vi "GDX_GetSensorInfo.vi"() -> (2 "battery level":u8)   [LabVIEW 2019]
uses:
  <vilib>/Vernier/GDX/GDX Controls/D2PIO_CHARGER_STATE.ctl
panel:
  out "Channel 15":i8
  out "Ch is Active 15":bool
  out "Channel Unit 15":string
  out "Channel Description 15":string
  out "Channel 14":i8
  out "Ch is Active 14":bool
  out "Channel Unit 14":string
  out "Channel Description 14":string
  out "Channel 13":i8
  out "Ch is Active 13":bool
  out "Channel Unit 13":string
  out "Channel Description 13":string
  out "Channel 12":i8
  out "Ch is Active 12":bool
  out "Channel Unit 12":string
  out "Channel Description 12":string
  out "Channel 11":i8
  out "Ch is Active 11":bool
  out "Channel Unit 11":string
  out "Channel Description 11":string
  out "Channel 10":i8
  out "Ch is Active 10":bool
  out "Channel Unit 10":string
  out "Channel Description 10":string
  out "Channel 9":i8
  out "Ch is Active 9":bool
  out "Channel Unit 9":string
  out "Channel Description 9":string
  out "Channel 8":i8
  out "Ch is Active 8":bool
  out "Channel Unit 8":string
  out "Channel Description 8":string
  out "Channel 7":i8
  out "Ch is Active 7":bool
  out "Channel Unit 7":string
  out "Channel Description 7":string
  out "Channel 6":i8
  out "Ch is Active 6":bool
  out "Channel Unit 6":string
  out "Channel Description 6":string
  out "Channel 5":i8
  out "Ch is Active 5":bool
  out "Channel Unit 5":string
  out "Channel Description 5":string
  out "Channel 4":i8
  out "Ch is Active 4":bool
  out "Channel Unit 4":string
  out "Channel Description 4":string
  out "Channel 3":i8
  out "Ch is Active 3":bool
  out "Channel Unit 3":string
  out "Channel Description 3":string
  out "Channel Unit 2":string
  out "Channel Description 2":string
  out "Ch is Active 2":bool
  out "Channel 2":i8
  out "Channel Unit":string
  out "Channel Description":string
  out "Ch is Active":bool
  out "Channel":i8
  out "BT Address (hex string)":string
  out "BLE Firmware (Numeric)":dbl
  out "DAQ Firmware (Numeric)":dbl
  out "Day":u8
  out "Month":u8
  out "Year":u16
  out "Device Name":string
  out "Device Friendly Name":string
  out "Serial Number":string
  out "Order Code":string
  out "CHARGER_STATE":T1 items=["IDLE", "CHARGING", "COMPLETE", "ERROR"]
  out "Available Channels":i8[](array[numeric])
  out "error out":errorcluster
  # "CHANNEL INFORMATION"
  # "DEVICE INFORMATION"
  # "Channel"
  # "Active?"
  # "Description"
  # "Unit"
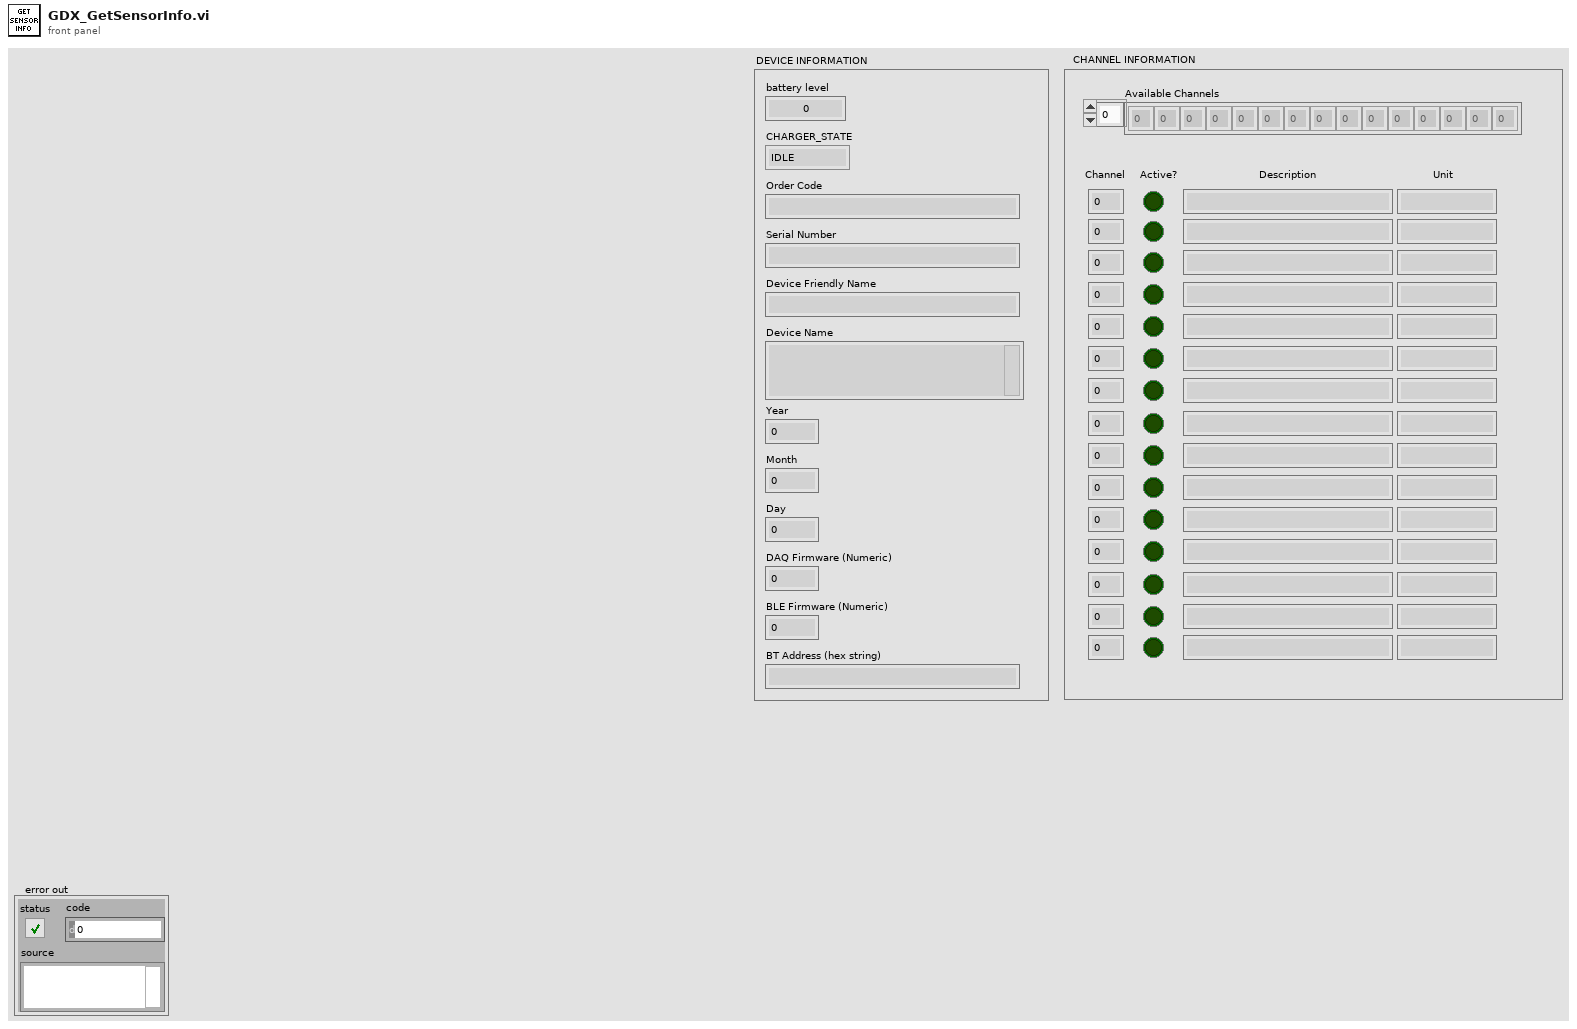
[diagram p1: front panel]
types:
  T1 = typedef "D2PIO_CHARGER_STATE.ctl" = u8
  T2 = typedef "D2PIO_D2PIOCluster.ctl" = cluster{"Library Handle":i64, "Device List Handle":i64, "BT Device Handles":i64[], "USB Device Handles":i64[], "BT+USB Device Handles":i64[], "Measurement Tick":dbl[], "Ch Availability Mask":u32[]}
  T3 = typedef "D2PIO_ChannelInfoCluster.ctl" = cluster{"Channel":i8, "Ch is Active":bool, "Channel ID":u32, "Channel Description":string, "Channel Unit":string}[]
  T4 = typedef "D2PIO_INFO_DeviceInfoCluster.ctl" = cluster{"battery level":u8, "CHARGER_STATE":T1, "Order Code":string, "Serial Number":string, "MFG ID":i16, "Device Friendly Name":string, "Device Name":string, "Year":u16, "Month":u8, "Day":u8, "DAQ Firmware (Numeric)":dbl, "DAQ Firmware (String)":string, "BLE Firmware (Numeric)":dbl, "BLE Firmware (String)":string, "BT Address (hex string)":string}
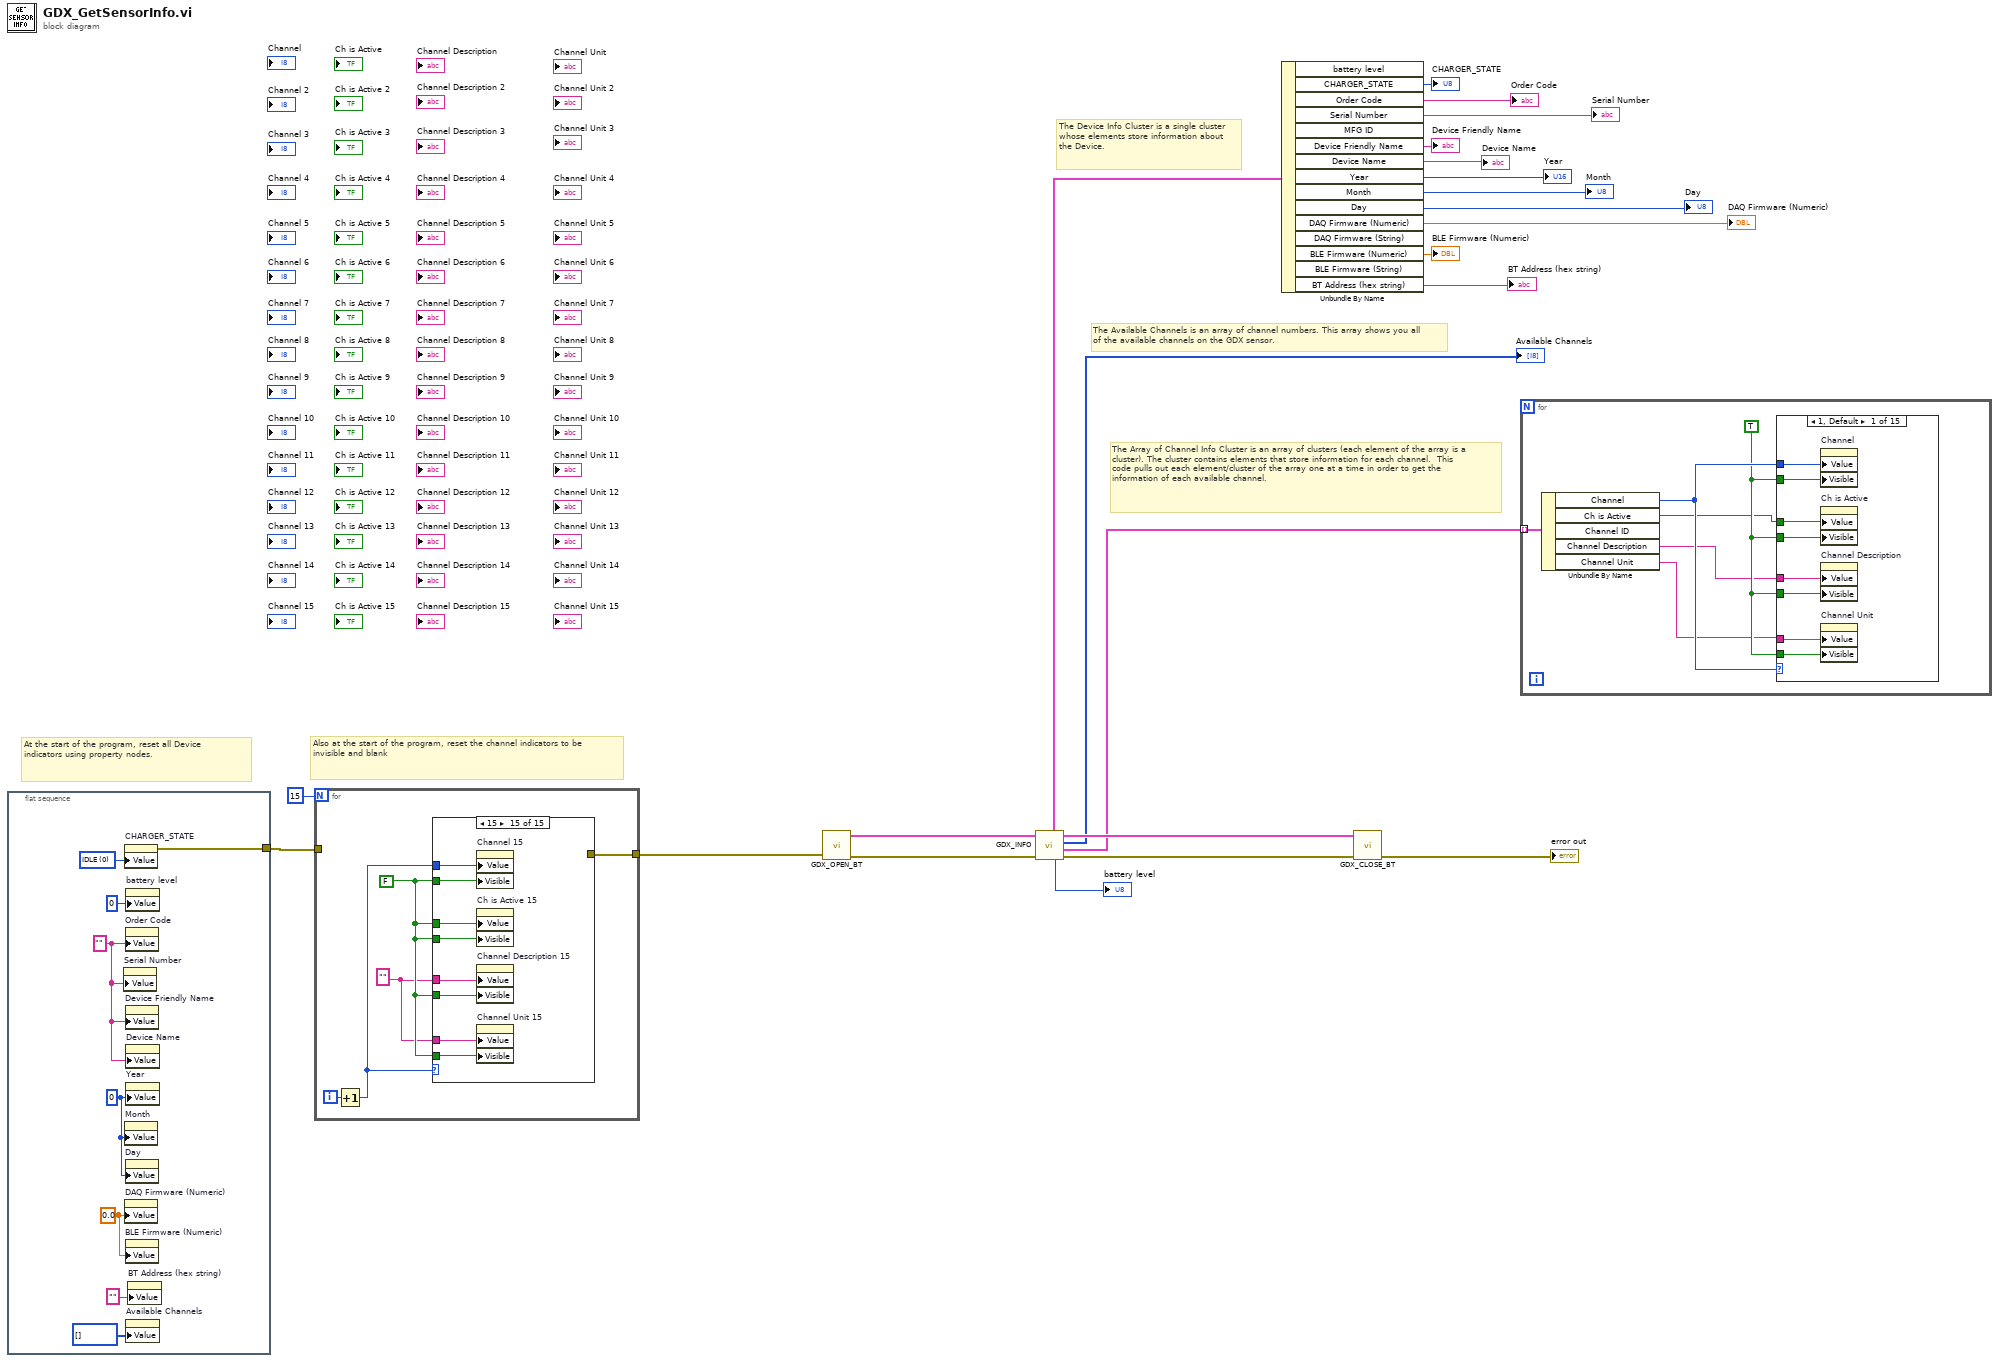
[diagram p0: block diagram]
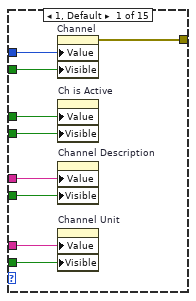
[diagram p2: hidden frame]
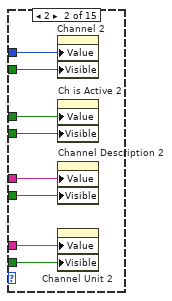
[diagram p3: hidden frame]
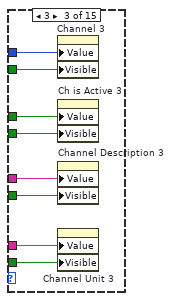
[diagram p4: hidden frame]
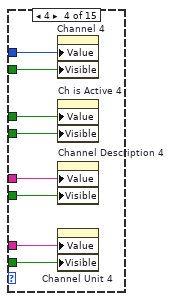
[diagram p5: hidden frame]
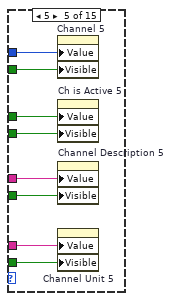
[diagram p6: hidden frame]
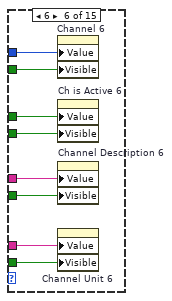
[diagram p7: hidden frame]
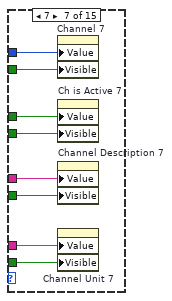
[diagram p8: hidden frame]
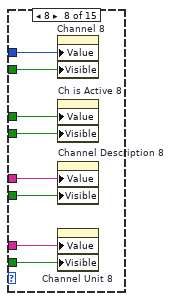
[diagram p9: hidden frame]
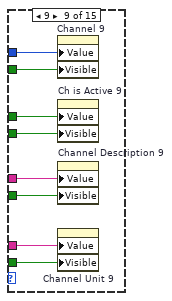
[diagram p10: hidden frame]
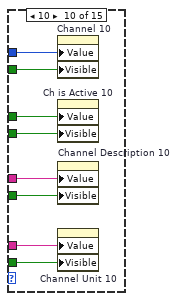
[diagram p11: hidden frame]
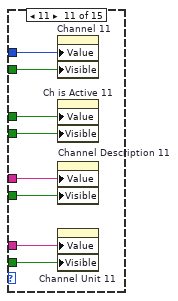
[diagram p12: hidden frame]
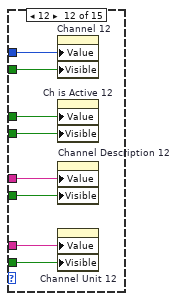
[diagram p13: hidden frame]
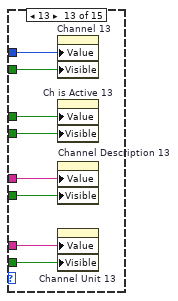
[diagram p14: hidden frame]
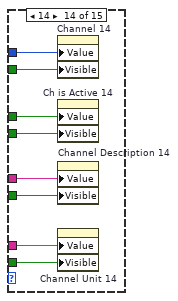
[diagram p15: hidden frame]
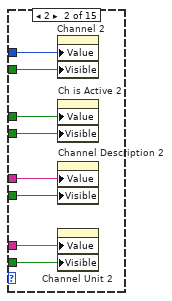
[diagram p16: hidden frame]
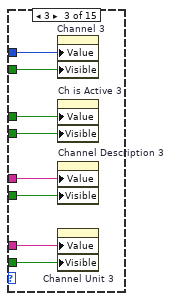
[diagram p17: hidden frame]
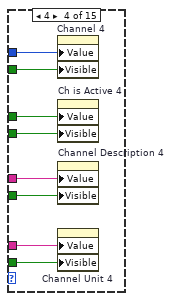
[diagram p18: hidden frame]
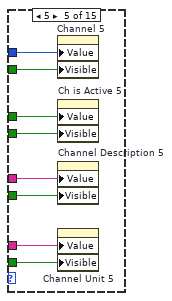
[diagram p19: hidden frame]
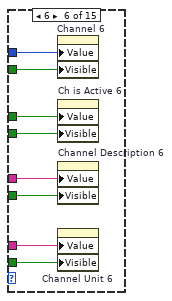
[diagram p20: hidden frame]
diagram:
  # "The Available Channels is an array of channel numbers. This array shows you all of the available channels on the GDX sensor."
  # "The Device Info Cluster is a single cluster whose elements store information about the Device."
  # "At the start of the program, reset all Device indicators using property nodes."
  # "The Array of Channel Info Cluster is an array of clusters (each element of the array is a cluster). The cluster contains elements that store information for each channel.  This code pulls out each element/cluster of the array one at a time in order to get the information of each available channel."
  # "Also at the start of the program, reset the channel indicators to be invisible and blank"
  n1 = flat-sequence {
    tunnel: [w25] -> w1
    frame #0 {
      w28 = 0.0 ("DAQ Firmware (Numeric)")
      w29 = u16 0 ("Year")
      w30 = "" ("Order Code")
      w31 = T1 0 items=["IDLE", "CHARGING", "COMPLETE", "ERROR"] ("CHARGER_STATE")
      n2 = property on="Serial Number" class="Str"("Value"=w30) -> ()  [unwired: 2 in, 2 out]
      n3 = property on="CHARGER_STATE" class="Ring (strict)"("Value"=w31) -> (error out=w25:errorcluster)  [unwired: 2 in, 1 out]
      n4 = property on="Month" class="DigNum (strict)"("Value"=w29) -> ()  [unwired: 2 in, 2 out]
      n5 = property on="DAQ Firmware (Numeric)" class="DigNum (strict)"("Value"=w28) -> ()  [unwired: 2 in, 2 out]
      n6 = property on="Order Code" class="Str"("Value"=w30) -> ()  [unwired: 2 in, 2 out]
      n7 = property on="Device Friendly Name" class="Str"("Value"=w30) -> ()  [unwired: 2 in, 2 out]
      n8 = property on="Day" class="DigNum (strict)"("Value"=w29) -> ()  [unwired: 2 in, 2 out]
      n9 = property on="BLE Firmware (Numeric)" class="DigNum (strict)"("Value"=w28) -> ()  [unwired: 2 in, 2 out]
      n10 = property on="battery level" class="DigNum (strict)"("Value"=u8 0 ("battery level")) -> ()  [unwired: 2 in, 2 out]
      n11 = property on="Device Name" class="Str"("Value"=w30) -> ()  [unwired: 2 in, 2 out]
      n12 = property on="Year" class="DigNum (strict)"("Value"=w29) -> ()  [unwired: 2 in, 2 out]
      n13 = property on="Available Channels" class="Arr (strict)"("Value"=i8[] [] ("Available Channels")) -> ()  [unwired: 2 in, 2 out]
      n14 = property on="BT Address (hex string)" class="Str"("Value"="" ("BT Address (hex string)")) -> ()  [unwired: 2 in, 2 out]
    }
  }
  n15 = for {
    N: 15 -> [_]
    tunnel: [w33] -> w2
    tunnel: w1 -> [_]
    i -> [w36]
    w34 = "" ("Channel Description")
    w35 = FALSE ("Visible")
    n16 = Increment(x=w36) -> (x+1=w32:i32)
    n17 = case shown="15" w32 {
      tunnel: w32 -> [w45 w53 w61 w69 w77 w85 w93 w101 w109 w117 w125 w133 w141 w149 w157]
      tunnel: w35 -> [w44 w52 w60 w68 w76 w84 w92 w100 w108 w116 w124 w132 w140 w148 w156]
      tunnel: w35 -> [w43 w51 w59 w67 w75 w83 w91 w99 w107 w115 w123 w131 w139 w147 w155]
      tunnel: w35 -> [w42 w50 w58 w66 w74 w82 w90 w98 w106 w114 w122 w130 w138 w146 w154]
      tunnel: w35 -> [w41 w49 w57 w65 w73 w81 w89 w97 w105 w113 w121 w129 w137 w145 w153]
      tunnel: w35 -> [w40 w48 w56 w64 w72 w80 w88 w96 w104 w112 w120 w128 w136 w144 w152]
      tunnel: w34 -> [w39 w47 w55 w63 w71 w79 w87 w95 w103 w111 w119 w127 w135 w143 w151]
      tunnel: w34 -> [w38 w46 w54 w62 w70 w78 w86 w94 w102 w110 w118 w126 w134 w142 w150]
      tunnel: [w37 _ _ _ _ _ _ _ _ _ _ _ _ _ _] -> w33
      frame 1, Default {
        n18 = property on="Channel" class="DigNum (strict)"("Value"=w45, "Visible"=w44) -> (error out=w37:errorcluster)  [unwired: 2 in, 1 out]
        n19 = property on="Ch is Active" class="Bool (strict)"("Value"=w40, "Visible"=w43) -> ()  [unwired: 2 in, 2 out]
        n20 = property on="Channel Description" class="Str"("Value"=w39, "Visible"=w42) -> ()  [unwired: 2 in, 2 out]
        n21 = property on="Channel Unit" class="Str"("Value"=w38, "Visible"=w41) -> ()  [unwired: 2 in, 2 out]
      }
      frame 2 {
        n22 = property on="Channel 2" class="DigNum (strict)"("Value"=w53, "Visible"=w52) -> ()  [unwired: 2 in, 2 out]
        n23 = property on="Ch is Active 2" class="Bool (strict)"("Value"=w48, "Visible"=w51) -> ()  [unwired: 2 in, 2 out]
        n24 = property on="Channel Description 2" class="Str"("Value"=w47, "Visible"=w50) -> ()  [unwired: 2 in, 2 out]
        n25 = property on="Channel Unit 2" class="Str"("Value"=w46, "Visible"=w49) -> ()  [unwired: 2 in, 2 out]
      }
      frame 3 {
        n26 = property on="Channel 3" class="DigNum (strict)"("Value"=w61, "Visible"=w60) -> ()  [unwired: 2 in, 2 out]
        n27 = property on="Ch is Active 3" class="Bool (strict)"("Value"=w56, "Visible"=w59) -> ()  [unwired: 2 in, 2 out]
        n28 = property on="Channel Description 3" class="Str"("Value"=w55, "Visible"=w58) -> ()  [unwired: 2 in, 2 out]
        n29 = property on="Channel Unit 3" class="Str"("Value"=w54, "Visible"=w57) -> ()  [unwired: 2 in, 2 out]
      }
      frame 4 {
        n30 = property on="Channel 4" class="DigNum (strict)"("Value"=w69, "Visible"=w68) -> ()  [unwired: 2 in, 2 out]
        n31 = property on="Ch is Active 4" class="Bool (strict)"("Value"=w64, "Visible"=w67) -> ()  [unwired: 2 in, 2 out]
        n32 = property on="Channel Description 4" class="Str"("Value"=w63, "Visible"=w66) -> ()  [unwired: 2 in, 2 out]
        n33 = property on="Channel Unit 4" class="Str"("Value"=w62, "Visible"=w65) -> ()  [unwired: 2 in, 2 out]
      }
      frame 5 {
        n34 = property on="Channel 5" class="DigNum (strict)"("Value"=w77, "Visible"=w76) -> ()  [unwired: 2 in, 2 out]
        n35 = property on="Ch is Active 5" class="Bool (strict)"("Value"=w72, "Visible"=w75) -> ()  [unwired: 2 in, 2 out]
        n36 = property on="Channel Description 5" class="Str"("Value"=w71, "Visible"=w74) -> ()  [unwired: 2 in, 2 out]
        n37 = property on="Channel Unit 5" class="Str"("Value"=w70, "Visible"=w73) -> ()  [unwired: 2 in, 2 out]
      }
      frame 6 {
        n38 = property on="Channel 6" class="DigNum (strict)"("Value"=w85, "Visible"=w84) -> ()  [unwired: 2 in, 2 out]
        n39 = property on="Ch is Active 6" class="Bool (strict)"("Value"=w80, "Visible"=w83) -> ()  [unwired: 2 in, 2 out]
        n40 = property on="Channel Description 6" class="Str"("Value"=w79, "Visible"=w82) -> ()  [unwired: 2 in, 2 out]
        n41 = property on="Channel Unit 6" class="Str"("Value"=w78, "Visible"=w81) -> ()  [unwired: 2 in, 2 out]
      }
      frame 7 {
        n42 = property on="Channel 7" class="DigNum (strict)"("Value"=w93, "Visible"=w92) -> ()  [unwired: 2 in, 2 out]
        n43 = property on="Ch is Active 7" class="Bool (strict)"("Value"=w88, "Visible"=w91) -> ()  [unwired: 2 in, 2 out]
        n44 = property on="Channel Description 7" class="Str"("Value"=w87, "Visible"=w90) -> ()  [unwired: 2 in, 2 out]
        n45 = property on="Channel Unit 7" class="Str"("Value"=w86, "Visible"=w89) -> ()  [unwired: 2 in, 2 out]
      }
      frame 8 {
        n46 = property on="Channel 8" class="DigNum (strict)"("Value"=w101, "Visible"=w100) -> ()  [unwired: 2 in, 2 out]
        n47 = property on="Ch is Active 8" class="Bool (strict)"("Value"=w96, "Visible"=w99) -> ()  [unwired: 2 in, 2 out]
        n48 = property on="Channel Description 8" class="Str"("Value"=w95, "Visible"=w98) -> ()  [unwired: 2 in, 2 out]
        n49 = property on="Channel Unit 8" class="Str"("Value"=w94, "Visible"=w97) -> ()  [unwired: 2 in, 2 out]
      }
      frame 9 {
        n50 = property on="Channel 9" class="DigNum (strict)"("Value"=w109, "Visible"=w108) -> ()  [unwired: 2 in, 2 out]
        n51 = property on="Ch is Active 9" class="Bool (strict)"("Value"=w104, "Visible"=w107) -> ()  [unwired: 2 in, 2 out]
        n52 = property on="Channel Description 9" class="Str"("Value"=w103, "Visible"=w106) -> ()  [unwired: 2 in, 2 out]
        n53 = property on="Channel Unit 9" class="Str"("Value"=w102, "Visible"=w105) -> ()  [unwired: 2 in, 2 out]
      }
      frame 10 {
        n54 = property on="Channel 10" class="DigNum (strict)"("Value"=w117, "Visible"=w116) -> ()  [unwired: 2 in, 2 out]
        n55 = property on="Ch is Active 10" class="Bool (strict)"("Value"=w112, "Visible"=w115) -> ()  [unwired: 2 in, 2 out]
        n56 = property on="Channel Description 10" class="Str"("Value"=w111, "Visible"=w114) -> ()  [unwired: 2 in, 2 out]
        n57 = property on="Channel Unit 10" class="Str"("Value"=w110, "Visible"=w113) -> ()  [unwired: 2 in, 2 out]
      }
      frame 11 {
        n58 = property on="Channel 11" class="DigNum (strict)"("Value"=w125, "Visible"=w124) -> ()  [unwired: 2 in, 2 out]
        n59 = property on="Ch is Active 11" class="Bool (strict)"("Value"=w120, "Visible"=w123) -> ()  [unwired: 2 in, 2 out]
        n60 = property on="Channel Description 11" class="Str"("Value"=w119, "Visible"=w122) -> ()  [unwired: 2 in, 2 out]
        n61 = property on="Channel Unit 11" class="Str"("Value"=w118, "Visible"=w121) -> ()  [unwired: 2 in, 2 out]
      }
      frame 12 {
        n62 = property on="Channel 12" class="DigNum (strict)"("Value"=w133, "Visible"=w132) -> ()  [unwired: 2 in, 2 out]
        n63 = property on="Ch is Active 12" class="Bool (strict)"("Value"=w128, "Visible"=w131) -> ()  [unwired: 2 in, 2 out]
        n64 = property on="Channel Description 12" class="Str"("Value"=w127, "Visible"=w130) -> ()  [unwired: 2 in, 2 out]
        n65 = property on="Channel Unit 12" class="Str"("Value"=w126, "Visible"=w129) -> ()  [unwired: 2 in, 2 out]
      }
      frame 13 {
        n66 = property on="Channel 13" class="DigNum (strict)"("Value"=w141, "Visible"=w140) -> ()  [unwired: 2 in, 2 out]
        n67 = property on="Ch is Active 13" class="Bool (strict)"("Value"=w136, "Visible"=w139) -> ()  [unwired: 2 in, 2 out]
        n68 = property on="Channel Description 13" class="Str"("Value"=w135, "Visible"=w138) -> ()  [unwired: 2 in, 2 out]
        n69 = property on="Channel Unit 13" class="Str"("Value"=w134, "Visible"=w137) -> ()  [unwired: 2 in, 2 out]
      }
      frame 14 {
        n70 = property on="Channel 14" class="DigNum (strict)"("Value"=w149, "Visible"=w148) -> ()  [unwired: 2 in, 2 out]
        n71 = property on="Ch is Active 14" class="Bool (strict)"("Value"=w144, "Visible"=w147) -> ()  [unwired: 2 in, 2 out]
        n72 = property on="Channel Description 14" class="Str"("Value"=w143, "Visible"=w146) -> ()  [unwired: 2 in, 2 out]
        n73 = property on="Channel Unit 14" class="Str"("Value"=w142, "Visible"=w145) -> ()  [unwired: 2 in, 2 out]
      }
      frame 15 {
        n74 = property on="Channel 15" class="DigNum (strict)"("Value"=w157, "Visible"=w156) -> ()  [unwired: 2 in, 2 out]
        n75 = property on="Ch is Active 15" class="Bool (strict)"("Value"=w152, "Visible"=w155) -> ()  [unwired: 2 in, 2 out]
        n76 = property on="Channel Description 15" class="Str"("Value"=w151, "Visible"=w154) -> ()  [unwired: 2 in, 2 out]
        n77 = property on="Channel Unit 15" class="Str"("Value"=w150, "Visible"=w153) -> ()  [unwired: 2 in, 2 out]
      }
    }
  }
  n78 = call <vilib>:"GDX_OPEN_BT.vi"("error in (no error)"=w2) -> ("error out"=w21:errorcluster, "D2PIO Cluster Out"=w22:T2)  [unwired: 9 in]
  n79 = call <vilib>:"GDX_INFO.vi"("error in (no error)"=w21, "D2PIO Cluster In"=w22) -> ("error out"=w19:errorcluster, "Array of Channel Info Cluster"=w4:T3, "Available Channels"=→"Available Channels":i8[], "D2PIO Cluster Out"=w20:T2, "battery level"=→"battery level":u8, "Device Info Cluster"=w16:T4)  [unwired: 4 in]
  n80 = Unbundle By Name(w16) -> ("CHARGER_STATE"=→"CHARGER_STATE":T1, "Order Code"=→"Order Code":string, "Serial Number"=→"Serial Number":string, "Device Friendly Name"=→"Device Friendly Name":string, "Device Name"=→"Device Name":string, "Year"=→"Year":u16, "Month"=→"Month":u8, "Day"=→"Day":u8, "DAQ Firmware (Numeric)"=→"DAQ Firmware (Numeric)":dbl, "BLE Firmware (Numeric)"=→"BLE Firmware (Numeric)":dbl, "BT Address (hex string)"=→"BT Address (hex string)":string)  [unwired: 4 out]
  n81 = call <vilib>:"GDX_CLOSE_BT.vi"("error in (no error)"=w19, "D2PIO Cluster In"=w20) -> ("error out"=→"error out":errorcluster)  [unwired: 8 in, 1 out]
  n82 = for {
    tunnel: w4 -> [w163] mode=indexing
    w161 = TRUE ("Visible")
    n83 = Unbundle By Name(w163) -> ("Channel"=w162:i8, "Ch is Active"=w160:bool, "Channel Description"=w159:string, "Channel Unit"=w158:string)  [unwired: 1 out]
    n84 = case shown="1, Default" w162 {
      tunnel: w162 -> [w171 w179 w187 w195 w203 w211 w219 w227 w235 w243 w251 w259 w267 w275 w283]
      tunnel: w161 -> [w170 w178 w186 w194 w202 w210 w218 w226 w234 w242 w250 w258 w266 w274 w282]
      tunnel: w161 -> [w169 w177 w185 w193 w201 w209 w217 w225 w233 w241 w249 w257 w265 w273 w281]
      tunnel: w161 -> [w168 w176 w184 w192 w200 w208 w216 w224 w232 w240 w248 w256 w264 w272 w280]
      tunnel: w161 -> [w167 w175 w183 w191 w199 w207 w215 w223 w231 w239 w247 w255 w263 w271 w279]
      tunnel: w160 -> [w166 w174 w182 w190 w198 w206 w214 w222 w230 w238 w246 w254 w262 w270 w278]
      tunnel: w159 -> [w165 w173 w181 w189 w197 w205 w213 w221 w229 w237 w245 w253 w261 w269 w277]
      tunnel: w158 -> [w164 w172 w180 w188 w196 w204 w212 w220 w228 w236 w244 w252 w260 w268 w276]
      frame 1, Default {
        n85 = property on="Channel" class="DigNum (strict)"("Value"=w171, "Visible"=w170) -> ()  [unwired: 2 in, 2 out]
        n86 = property on="Ch is Active" class="Bool (strict)"("Value"=w166, "Visible"=w169) -> ()  [unwired: 2 in, 2 out]
        n87 = property on="Channel Description" class="Str"("Value"=w165, "Visible"=w168) -> ()  [unwired: 2 in, 2 out]
        n88 = property on="Channel Unit" class="Str"("Value"=w164, "Visible"=w167) -> ()  [unwired: 2 in, 2 out]
      }
      frame 2 {
        n89 = property on="Channel 2" class="DigNum (strict)"("Value"=w179, "Visible"=w178) -> ()  [unwired: 2 in, 2 out]
        n90 = property on="Ch is Active 2" class="Bool (strict)"("Value"=w174, "Visible"=w177) -> ()  [unwired: 2 in, 2 out]
        n91 = property on="Channel Description 2" class="Str"("Value"=w173, "Visible"=w176) -> ()  [unwired: 2 in, 2 out]
        n92 = property on="Channel Unit 2" class="Str"("Value"=w172, "Visible"=w175) -> ()  [unwired: 2 in, 2 out]
      }
      frame 3 {
        n93 = property on="Channel 3" class="DigNum (strict)"("Value"=w187, "Visible"=w186) -> ()  [unwired: 2 in, 2 out]
        n94 = property on="Ch is Active 3" class="Bool (strict)"("Value"=w182, "Visible"=w185) -> ()  [unwired: 2 in, 2 out]
        n95 = property on="Channel Description 3" class="Str"("Value"=w181, "Visible"=w184) -> ()  [unwired: 2 in, 2 out]
        n96 = property on="Channel Unit 3" class="Str"("Value"=w180, "Visible"=w183) -> ()  [unwired: 2 in, 2 out]
      }
      frame 4 {
        n97 = property on="Channel 4" class="DigNum (strict)"("Value"=w195, "Visible"=w194) -> ()  [unwired: 2 in, 2 out]
        n98 = property on="Ch is Active 4" class="Bool (strict)"("Value"=w190, "Visible"=w193) -> ()  [unwired: 2 in, 2 out]
        n99 = property on="Channel Description 4" class="Str"("Value"=w189, "Visible"=w192) -> ()  [unwired: 2 in, 2 out]
        n100 = property on="Channel Unit 4" class="Str"("Value"=w188, "Visible"=w191) -> ()  [unwired: 2 in, 2 out]
      }
      frame 5 {
        n101 = property on="Channel 5" class="DigNum (strict)"("Value"=w203, "Visible"=w202) -> ()  [unwired: 2 in, 2 out]
        n102 = property on="Ch is Active 5" class="Bool (strict)"("Value"=w198, "Visible"=w201) -> ()  [unwired: 2 in, 2 out]
        n103 = property on="Channel Description 5" class="Str"("Value"=w197, "Visible"=w200) -> ()  [unwired: 2 in, 2 out]
        n104 = property on="Channel Unit 5" class="Str"("Value"=w196, "Visible"=w199) -> ()  [unwired: 2 in, 2 out]
      }
      frame 6 {
        n105 = property on="Channel 6" class="DigNum (strict)"("Value"=w211, "Visible"=w210) -> ()  [unwired: 2 in, 2 out]
        n106 = property on="Ch is Active 6" class="Bool (strict)"("Value"=w206, "Visible"=w209) -> ()  [unwired: 2 in, 2 out]
        n107 = property on="Channel Description 6" class="Str"("Value"=w205, "Visible"=w208) -> ()  [unwired: 2 in, 2 out]
        n108 = property on="Channel Unit 6" class="Str"("Value"=w204, "Visible"=w207) -> ()  [unwired: 2 in, 2 out]
      }
      frame 7 {
        n109 = property on="Channel 7" class="DigNum (strict)"("Value"=w219, "Visible"=w218) -> ()  [unwired: 2 in, 2 out]
        n110 = property on="Ch is Active 7" class="Bool (strict)"("Value"=w214, "Visible"=w217) -> ()  [unwired: 2 in, 2 out]
        n111 = property on="Channel Description 7" class="Str"("Value"=w213, "Visible"=w216) -> ()  [unwired: 2 in, 2 out]
        n112 = property on="Channel Unit 7" class="Str"("Value"=w212, "Visible"=w215) -> ()  [unwired: 2 in, 2 out]
      }
      frame 8 {
        n113 = property on="Channel 8" class="DigNum (strict)"("Value"=w227, "Visible"=w226) -> ()  [unwired: 2 in, 2 out]
        n114 = property on="Ch is Active 8" class="Bool (strict)"("Value"=w222, "Visible"=w225) -> ()  [unwired: 2 in, 2 out]
        n115 = property on="Channel Description 8" class="Str"("Value"=w221, "Visible"=w224) -> ()  [unwired: 2 in, 2 out]
        n116 = property on="Channel Unit 8" class="Str"("Value"=w220, "Visible"=w223) -> ()  [unwired: 2 in, 2 out]
      }
      frame 9 {
        n117 = property on="Channel 9" class="DigNum (strict)"("Value"=w235, "Visible"=w234) -> ()  [unwired: 2 in, 2 out]
        n118 = property on="Ch is Active 9" class="Bool (strict)"("Value"=w230, "Visible"=w233) -> ()  [unwired: 2 in, 2 out]
        n119 = property on="Channel Description 9" class="Str"("Value"=w229, "Visible"=w232) -> ()  [unwired: 2 in, 2 out]
        n120 = property on="Channel Unit 9" class="Str"("Value"=w228, "Visible"=w231) -> ()  [unwired: 2 in, 2 out]
      }
      frame 10 {
        n121 = property on="Channel 10" class="DigNum (strict)"("Value"=w243, "Visible"=w242) -> ()  [unwired: 2 in, 2 out]
        n122 = property on="Ch is Active 10" class="Bool (strict)"("Value"=w238, "Visible"=w241) -> ()  [unwired: 2 in, 2 out]
        n123 = property on="Channel Description 10" class="Str"("Value"=w237, "Visible"=w240) -> ()  [unwired: 2 in, 2 out]
        n124 = property on="Channel Unit 10" class="Str"("Value"=w236, "Visible"=w239) -> ()  [unwired: 2 in, 2 out]
      }
      frame 11 {
        n125 = property on="Channel 11" class="DigNum (strict)"("Value"=w251, "Visible"=w250) -> ()  [unwired: 2 in, 2 out]
        n126 = property on="Ch is Active 11" class="Bool (strict)"("Value"=w246, "Visible"=w249) -> ()  [unwired: 2 in, 2 out]
        n127 = property on="Channel Description 11" class="Str"("Value"=w245, "Visible"=w248) -> ()  [unwired: 2 in, 2 out]
        n128 = property on="Channel Unit 11" class="Str"("Value"=w244, "Visible"=w247) -> ()  [unwired: 2 in, 2 out]
      }
      frame 12 {
        n129 = property on="Channel 12" class="DigNum (strict)"("Value"=w259, "Visible"=w258) -> ()  [unwired: 2 in, 2 out]
        n130 = property on="Ch is Active 12" class="Bool (strict)"("Value"=w254, "Visible"=w257) -> ()  [unwired: 2 in, 2 out]
        n131 = property on="Channel Description 12" class="Str"("Value"=w253, "Visible"=w256) -> ()  [unwired: 2 in, 2 out]
        n132 = property on="Channel Unit 12" class="Str"("Value"=w252, "Visible"=w255) -> ()  [unwired: 2 in, 2 out]
      }
      frame 13 {
        n133 = property on="Channel 13" class="DigNum (strict)"("Value"=w267, "Visible"=w266) -> ()  [unwired: 2 in, 2 out]
        n134 = property on="Ch is Active 13" class="Bool (strict)"("Value"=w262, "Visible"=w265) -> ()  [unwired: 2 in, 2 out]
        n135 = property on="Channel Description 13" class="Str"("Value"=w261, "Visible"=w264) -> ()  [unwired: 2 in, 2 out]
        n136 = property on="Channel Unit 13" class="Str"("Value"=w260, "Visible"=w263) -> ()  [unwired: 2 in, 2 out]
      }
      frame 14 {
        n137 = property on="Channel 14" class="DigNum (strict)"("Value"=w275, "Visible"=w274) -> ()  [unwired: 2 in, 2 out]
        n138 = property on="Ch is Active 14" class="Bool (strict)"("Value"=w270, "Visible"=w273) -> ()  [unwired: 2 in, 2 out]
        n139 = property on="Channel Description 14" class="Str"("Value"=w269, "Visible"=w272) -> ()  [unwired: 2 in, 2 out]
        n140 = property on="Channel Unit 14" class="Str"("Value"=w268, "Visible"=w271) -> ()  [unwired: 2 in, 2 out]
      }
      frame 15 {
        n141 = property on="Channel 15" class="DigNum (strict)"("Value"=w283, "Visible"=w282) -> ()  [unwired: 2 in, 2 out]
        n142 = property on="Ch is Active 15" class="Bool (strict)"("Value"=w278, "Visible"=w281) -> ()  [unwired: 2 in, 2 out]
        n143 = property on="Channel Description 15" class="Str"("Value"=w277, "Visible"=w280) -> ()  [unwired: 2 in, 2 out]
        n144 = property on="Channel Unit 15" class="Str"("Value"=w276, "Visible"=w279) -> ()  [unwired: 2 in, 2 out]
      }
    }
  }
